vi "Autonomous Recorder.vi"(8 "error in (no error)":errorcluster) -> ()   [LabVIEW 2011]
uses:
  Shared/Autonomous Recording TypeDef.ctl
  Shooter Global.vi
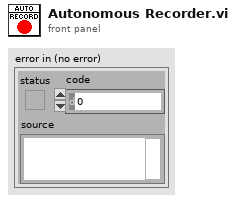
[diagram p1: front panel]
types:
  T1 = typedef "WPI_JoystickDevRef.ctl" = cluster{"Device":T2}
  T2 = typedef "WPI_JoystickDeviceEnum.ctl" = enum16{"USB 1", "USB 2", "USB 3", "USB 4", "Kinect 1", "Kinect 2"}
  T3 = enum16{"open", "replace", "create", "open or create", "replace or create", "replace or create with confirmation"}
  T4 = typedef "WPI_JoystickButtonState.ctl" = cluster{"Button 1":bool, "Button 2":bool, "Button 3":bool, "Button 4":bool, "Button 5":bool, "Button 6":bool, "Button 7":bool, "Button 8":bool, "Button 9":bool, "Button 10":bool, "Button 11":bool, "Button 12":bool}
  T5 = typedef "WPI_EncoderDevRef.ctl" = cluster{"DevStatus":errorcluster, "EncoderIndex":T6, "CounterIndex":T7, "DistancePerCount":dbl, "Decoding Type":T8}
  T6 = typedef "FPGA_EncoderIdx.ctl" = enum8{"Enc 0", "Enc 1", "Enc 2", "Enc 3", "Invalid"}
  T7 = typedef "FPGA_CounterCtrSystemIndex.ctl" = enum8{"Ctr 0", "Ctr 1", "Ctr 2", "Ctr 3", "Ctr 4", "Ctr 5", "Ctr 6", "Ctr 7", "Invalid"}
  T8 = typedef "WPI_EncoderType.ctl" = enum16{"1x", "2x", "4x"}
  T9 = typedef "Autonomous Recording TypeDef.ctl" = cluster{"Left Drive Encoder":dbl, "Right Drive Encoder":dbl, "Shooter Mode":enum16{"Off", "Open Loop Control", "Closed Loop Control", "Top Spin"}, "Set RPM":dbl, "Set Motor Speed":dbl, "Horn":bool, "Shift Low":bool, "Shift High":bool, "Fire":bool, "Reset Encoders":bool}
  T10 = enum16{"Off", "Open Loop Control", "Closed Loop Control", "Top Spin"}
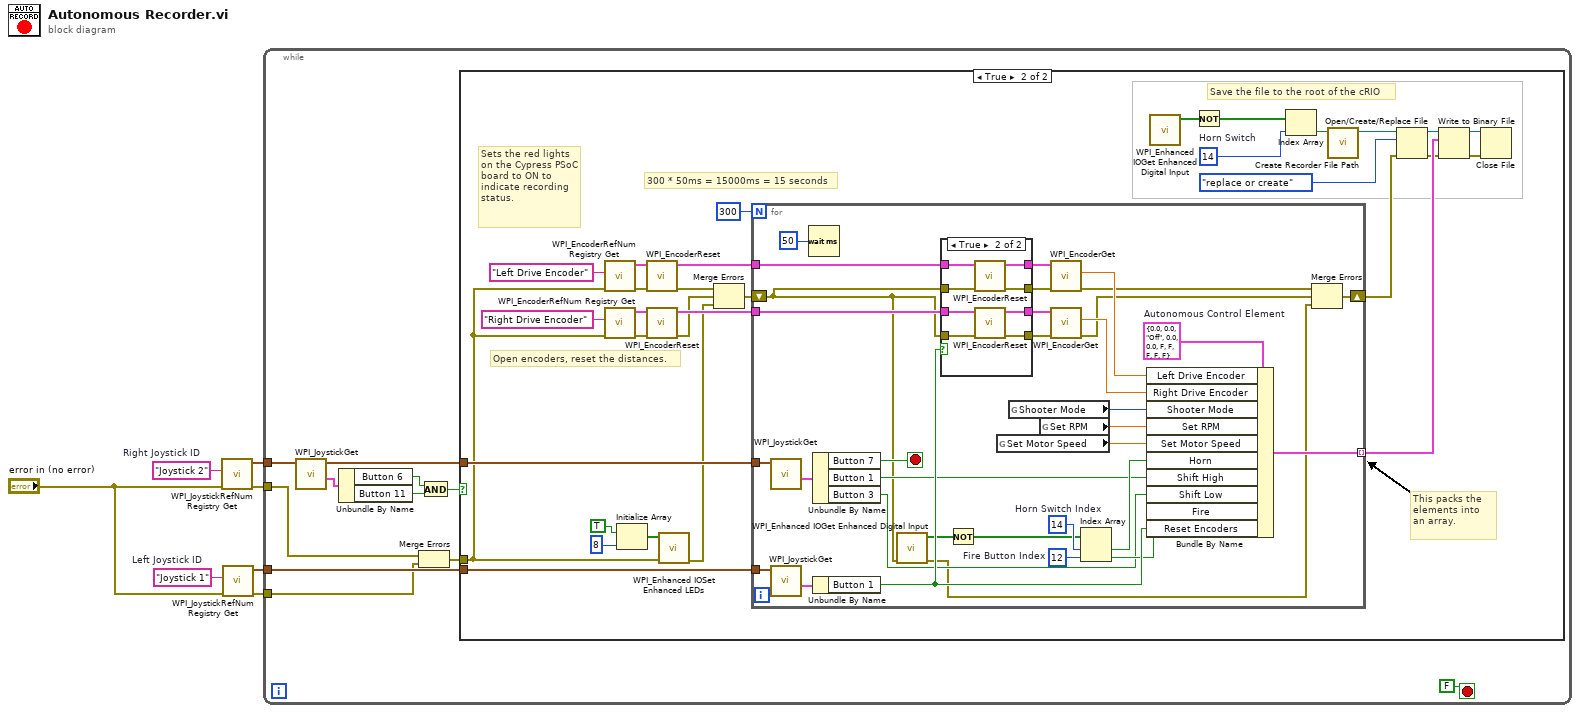
[diagram p0: block diagram]
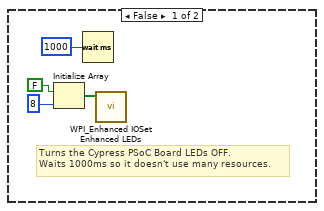
[diagram p2: hidden frame]
diagram:
  w5 = "Joystick 1"  # Left Joystick ID
  w4 = "Joystick 2"  # Right Joystick ID
  n1 = call <vilib>:"WPI_JoystickRefNum Registry Get.vi"("error in (no error)"="error in (no error)", "refnum name"=w4) -> ("error out"=w2:errorcluster, "JoystickDevRef"=w3:T1)  [unwired: 8 in]
  n2 = call <vilib>:"WPI_JoystickRefNum Registry Get.vi"("error in (no error)"="error in (no error)", "refnum name"=w5) -> ("error out"=w1:errorcluster, "JoystickDevRef"=w6:T1)  [unwired: 8 in]
  n3 = while {
    tunnel: w3 -> [w17]
    tunnel: w6 -> [w11]
    tunnel: w2 -> [w9]
    tunnel: w1 -> [w8]
    stop <- FALSE stop-if-true
    n4 = call <vilib>:"WPI_JoystickGet.vi"("JoystickDevRef"=w17) -> ("Buttons"=w15:T4, "JoystickDevRef"=w16:T1)  [unwired: 4 in, 1 out]
    n5 = Unbundle By Name(w15) -> ("Button 6"=w13:bool, "Button 11"=w14:bool)
    n6 = Merge Errors(w9, w8) -> (w10:errorcluster)
    n7 = And(x=w13, y=w14) -> (x .and. y?=w12:bool)
    n8 = case shown="True" w12 {
      tunnel: w16 -> [_ w45]
      tunnel: w11 -> [_ w36]
      tunnel: w10 -> [_ w28]
      frame False {
        # "Turns the Cypress PSoC Board LEDs OFF.\nWaits 1000ms so it doesn't use many resources."
        n9 = Initialize Array(FALSE ("element"), 8 ("dimension size")) -> (w22:bool[])
        n10 = Wait (ms)(milliseconds to wait=u32 1000) -> ()  [unwired: 1 out]
        n11 = call <vilib>:"WPI_Enhanced IOSet Enhanced LEDs.vi"("LEDs [1-8]"=w22) -> ()  [unwired: 10 in, 1 out]
      }
      frame True {
        w39 = 14  # Horn Switch
        # "Save the file to the root of the cRIO"
        # "300 * 50ms = 15000ms = 15 seconds"
        # "This packs the elements into\nan array."
        # "Sets the red lights on the Cypress PSoC board to ON to indicate recording status."
        # "Open encoders, reset the distances."
        n12 = call <vilib>:"WPI_EncoderRefNum Registry Get.vi"("error in (no error)"=w28, "refnum name"="Left Drive Encoder") -> ("error out"=w51:errorcluster, "EncoderDevRef"=w50:T5)  [unwired: 8 in]
        n13 = call <vilib>:"WPI_EncoderRefNum Registry Get.vi"("error in (no error)"=w28, "refnum name"="Right Drive Encoder") -> ("error out"=w49:errorcluster, "EncoderDevRef"=w48:T5)  [unwired: 8 in]
        n14 = Initialize Array(TRUE, 8 ("dimension size")) -> (w38:bool[])
        n15 = call <vilib>:"WPI_EncoderReset.vi"("error in (no error)"=w51, "EncoderDevRef"=w50) -> ("error out"=w25:errorcluster, "EncoderDevRef"=w47:T5)  [unwired: 8 out]
        n16 = call <vilib>:"WPI_EncoderReset.vi"("error in (no error)"=w49, "EncoderDevRef"=w48) -> ("error out"=w24:errorcluster, "EncoderDevRef"=w46:T5)  [unwired: 8 out]
        n17 = call <vilib>:"WPI_Enhanced IOSet Enhanced LEDs.vi"("error in (no error)"=w28, "LEDs [1-8]"=w38) -> ("error out"=w23:errorcluster)  [unwired: 9 in]
        n18 = Merge Errors(w25, w24, w23) -> (w26:errorcluster)
        n19 = for {
          N: 300 -> [_]
          tunnel: w47 -> [w76]
          tunnel: w46 -> [w75]
          tunnel: w45 -> [w85]
          tunnel: [w59] -> w31 mode=indexing
          tunnel: w36 -> [w70]
          shift-right: [w55] -> w27
          shift-left: w26 -> [w54]
          stop <- w82 stop-if-true
          w63 = 12  # Fire Button Index
          w67 = 14  # Horn Switch Index
          w83 = T9 {"Left Drive Encoder"=0.0, "Right Drive Encoder"=0.0, "Shooter Mode"=enum."Off", "Set RPM"=0.0, "Set Motor Speed"=0.0, "Horn"=FALSE, "Shift Low"=FALSE, "Shift High"=FALSE, "Fire"=FALSE, "Reset Encoders"=FALSE}  # Autonomous Control Element
          n20 = call <vilib>:"WPI_JoystickGet.vi"("JoystickDevRef"=w85) -> ("Buttons"=w84:T4)  [unwired: 4 in, 2 out]
          n21 = call <vilib>:"WPI_JoystickGet.vi"("JoystickDevRef"=w70) -> ("Buttons"=w69:T4)  [unwired: 4 in, 2 out]
          n22 = Wait (ms)(milliseconds to wait=u32 50) -> ()  [unwired: 1 out]
          n23 = Unbundle By Name(w84) -> ("Button 7"=w82:bool, "Button 1"=w61:bool, "Button 3"=w60:bool)
          n24 = Unbundle By Name(w69) -> ("Button 1"=w68:bool)
          n25 = call <vilib>:"WPI_Enhanced IOGet Enhanced Digital Input.vi"("error in (no error)"=w54) -> ("error out"=w56:errorcluster, "Digital Input [1-16]"=w65:bool[])  [unwired: 9 in]
          n26 = case shown="True" w68 {
            tunnel: w54 -> [w89 w98]
            tunnel: w76 -> [w90 w97]
            tunnel: w75 -> [w88 w96]
            tunnel: w54 -> [w87 w95]
            tunnel: [w90 w94] -> w74
            tunnel: [w89 w93] -> w73
            tunnel: [w88 w92] -> w72
            tunnel: [w87 w91] -> w71
            frame False {
            }
            frame True {
              n27 = call <vilib>:"WPI_EncoderReset.vi"("error in (no error)"=w98, "EncoderDevRef"=w97) -> ("error out"=w93:errorcluster, "EncoderDevRef"=w94:T5)  [unwired: 8 out]
              n28 = call <vilib>:"WPI_EncoderReset.vi"("error in (no error)"=w95, "EncoderDevRef"=w96) -> ("error out"=w91:errorcluster, "EncoderDevRef"=w92:T5)  [unwired: 8 out]
            }
          }
          n29 = Not(x=w65) -> (.not. x?=w64:bool[])
          n30 = global read "Shooter Global.vi" "Set Motor Speed"() -> (w78:dbl)
          n31 = global read "Shooter Global.vi" "Shooter Mode"() -> (w79:T10)
          n32 = global read "Shooter Global.vi" "Set RPM"() -> (w77:dbl)
          n33 = call <vilib>:"WPI_EncoderGet.vi"("error in (no error)"=w73, "EncoderDevRef"=w74) -> ("error out"=w58:errorcluster, "Distance"=w81:dbl)  [unwired: 8 out]
          n34 = call <vilib>:"WPI_EncoderGet.vi"("error in (no error)"=w71, "EncoderDevRef"=w72) -> ("error out"=w57:errorcluster, "Distance"=w80:dbl)  [unwired: 8 out]
          n35 = Index Array(array=w64, index #1=w67, index #2=w63) -> (element #1=w66:bool, element #2=w62:bool)
          n36 = Bundle By Name(cluster=w83, "Left Drive Encoder"=w81, "Right Drive Encoder"=w80, "Shooter Mode"=w79, "Set RPM"=w77, "Set Motor Speed"=w78, "Horn"=w66, "Shift High"=w61, "Shift Low"=w60, "Fire"=w62, "Reset Encoders"=w68) -> (w59:T9)
          n37 = Merge Errors(w58, w57, w56) -> (w55:errorcluster)
        }
        n38 = call <vilib>:"WPI_Enhanced IOGet Enhanced Digital Input.vi"() -> ("Digital Input [1-16]"=w43:bool[])  [unwired: 10 in, 1 out]
        n39 = Not(x=w43) -> (.not. x?=w44:bool[])
        n40 = Index Array(array=w44, index=w39) -> (element=w42:bool)
        n41 = call "Create Recorder File Path.vi"("T: Move_Shoot\nF: Shoot_Move"=w42) -> ("Path"=w35:path)  [unwired: 10 in]
        n42 = Open/Create/Replace File(file path (use dialog)=w35, error in=w27, operation (0:open)=T3."replace or create") -> (refnum out=w34:refnum<file>, error out=w30:errorcluster)  [unwired: 3 in, 1 out]
        n43 = Write to Binary File(file (use dialog)=w34, data=w31, error in=w30) -> (refnum out=w33:refnum<file>, error out=w32:errorcluster)  [unwired: 3 in, 1 out]
        n44 = Close File(refnum=w33, error in=w32) -> ()  [unwired: 2 out]
      }
    }
  }
